vi "background2.vi"() -> ()   [LabVIEW 2014]
uses:
  <vilib>/Utility/inputDevices.llb/keyboardAcquire.vi
  <vilib>/Utility/inputDevices.llb/closeKeyboard.vi
panel:
  out "1jump":bool=TRUE
  out "black hole":T1
  out "火右飛 2":bool=TRUE
  out "火左飛 2":bool
  out "火左飛":bool
  out "1":T2
  out "火右飛":bool=TRUE
  out "2":T3
  out "2-1":T2
  out "2-2":T3
  in  "stop jump2":bool
  out "Position:Top 2":i32
  out "Position:Left 2":i32
  in  "stop jump1":bool
  out "人1":T4
  out "keys pressed":T5(array[ring])
  in  "right/left 2":bool
  in  "人2":bool
  in  "right/left":bool
  in  "人1":bool
  out "人2":T4
  out "Position:Top":i32
  out "Position:Left":i32
  in  "stop":bool
  # "W:17\nS:31\nA:30\nD:32"
  # "上:72\n下:80\n左:75\n右:77"
  # "17"
  # "48"
  # "587"
  # "168"
  # "523"
  # "623"
  # "678"
  # "334"
  # "288"
  # "408"
  # "1049"
  # "212"
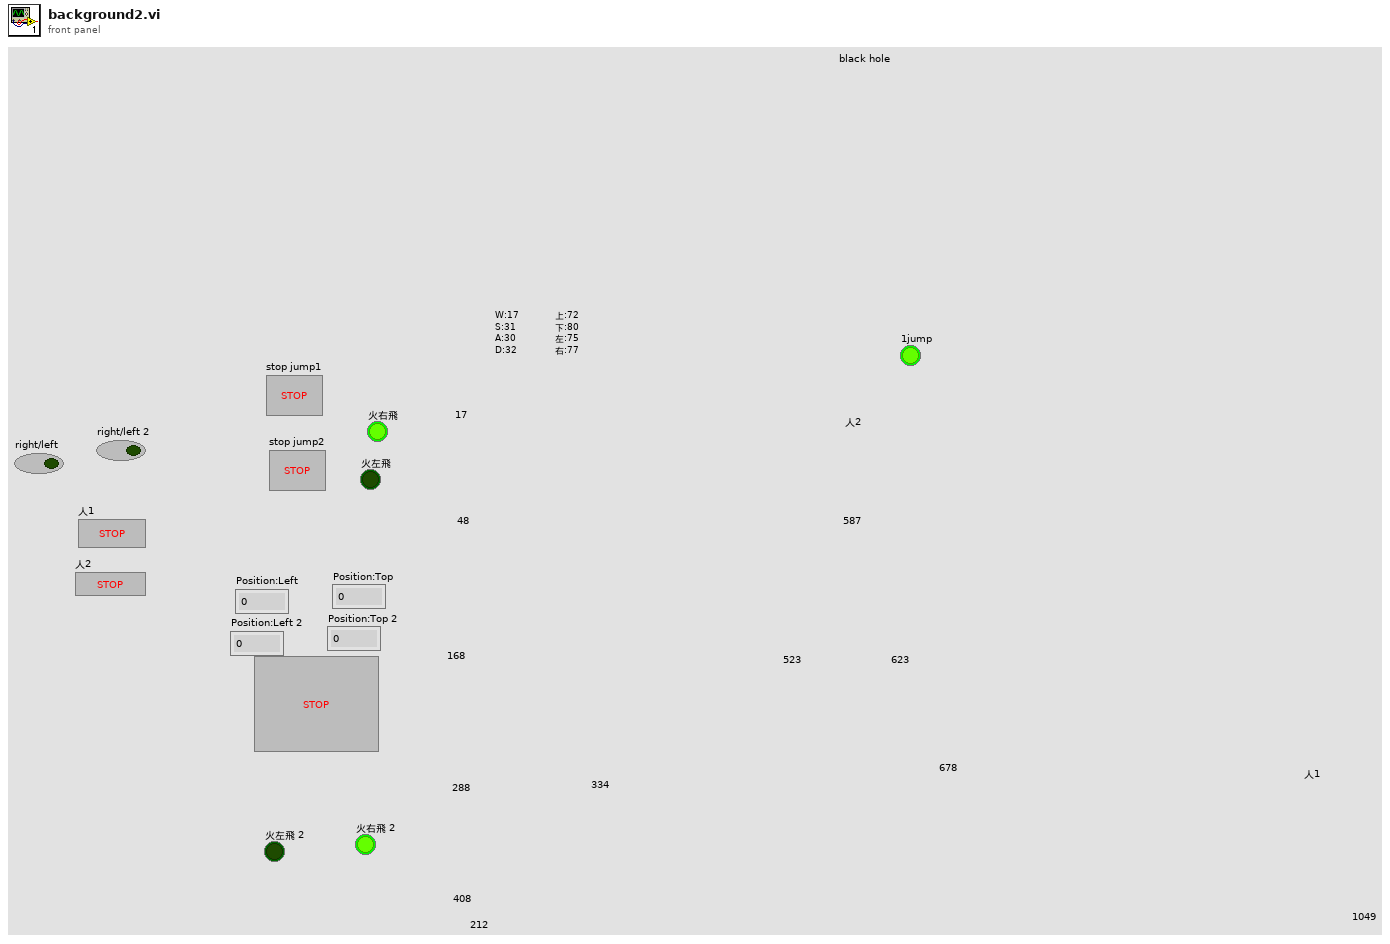
[diagram p1: front panel]
types:
  T1 = typedef "Control 4.ctl" = u16
  T2 = typedef "火焰.ctl" = u16
  T3 = typedef "火焰2.ctl" = u16
  T4 = typedef "Control 3.ctl" = u16
  T5 = enum16{"0", "1", "2", "3", "4", "5", "6", "7", "8", "9", "A", "B", "C", "D", "E", "F", "G", "H", "I", "J", "K", "L", "M", "N", "O", "P", "Q", "R", "S", "T", "U", "V", "W", "X", "Y", "Z", "F1", "F2", "F3", "F4", "F5", "F6", "F7", "F8", "F9", "F10", "F11", "F12", "F13", "F14", "F15", "ADD", "BACK", "BACKSLASH", "CAPITAL", "COMMA", "DECIMAL", "DELETE", "DIVIDE", "DOWN", "END", "EQUALS", "ESCAPE", "GRAVE (`)", "HOME", "INSERT", "LBRACKET", "LCONTROL", "LEFT", "L ALT", "LSHIFT", "LWIN", "MINUS", "MULTIPLY", "NEXT", "NUMLOCK", "NUMPAD_0", "NUMPAD_1", "NUMPAD_2", "NUMPAD_3", "NUMPAD_4", "NUMPAD_5", "NUMPAD_6", "NUMPAD_7", "NUMPAD_8", "NUMPAD_9", "PAUSE", "PERIOD", "PRIOR (PG UP)", "RBRACKET", "RCONTROL", "RETURN", "RIGHT", "R ALT", "RSHIFT", "RWIN", "SCROLL", "SEMICOLON", "SLASH", "SPACE", "SUBTRACT", "TAB", "UP", "ENTER (num pad)", "' (quote)"}[]
  T6 = enum16{"0", "1", "2", "3", "4", "5", "6", "7", "8", "9", "A", "B", "C", "D", "E", "F", "G", "H", "I", "J", "K", "L", "M", "N", "O", "P", "Q", "R", "S", "T", "U", "V", "W", "X", "Y", "Z", "F1", "F2", "F3", "F4", "F5", "F6", "F7", "F8", "F9", "F10", "F11", "F12", "F13", "F14", "F15", "ADD", "BACK", "BACKSLASH", "CAPITAL", "COMMA", "DECIMAL", "DELETE", "DIVIDE", "DOWN", "END", "EQUALS", "ESCAPE", "GRAVE (`)", "HOME", "INSERT", "LBRACKET", "LCONTROL", "LEFT", "L ALT", "LSHIFT", "LWIN", "MINUS", "MULTIPLY", "NEXT", "NUMLOCK", "NUMPAD_0", "NUMPAD_1", "NUMPAD_2", "NUMPAD_3", "NUMPAD_4", "NUMPAD_5", "NUMPAD_6", "NUMPAD_7", "NUMPAD_8", "NUMPAD_9", "PAUSE", "PERIOD", "PRIOR (PG UP)", "RBRACKET", "RCONTROL", "RETURN", "RIGHT", "R ALT", "RSHIFT", "RWIN", "SCROLL", "SEMICOLON", "SLASH", "SPACE", "SUBTRACT", "TAB", "UP", "ENTER (num pad)", "' (quote)"}
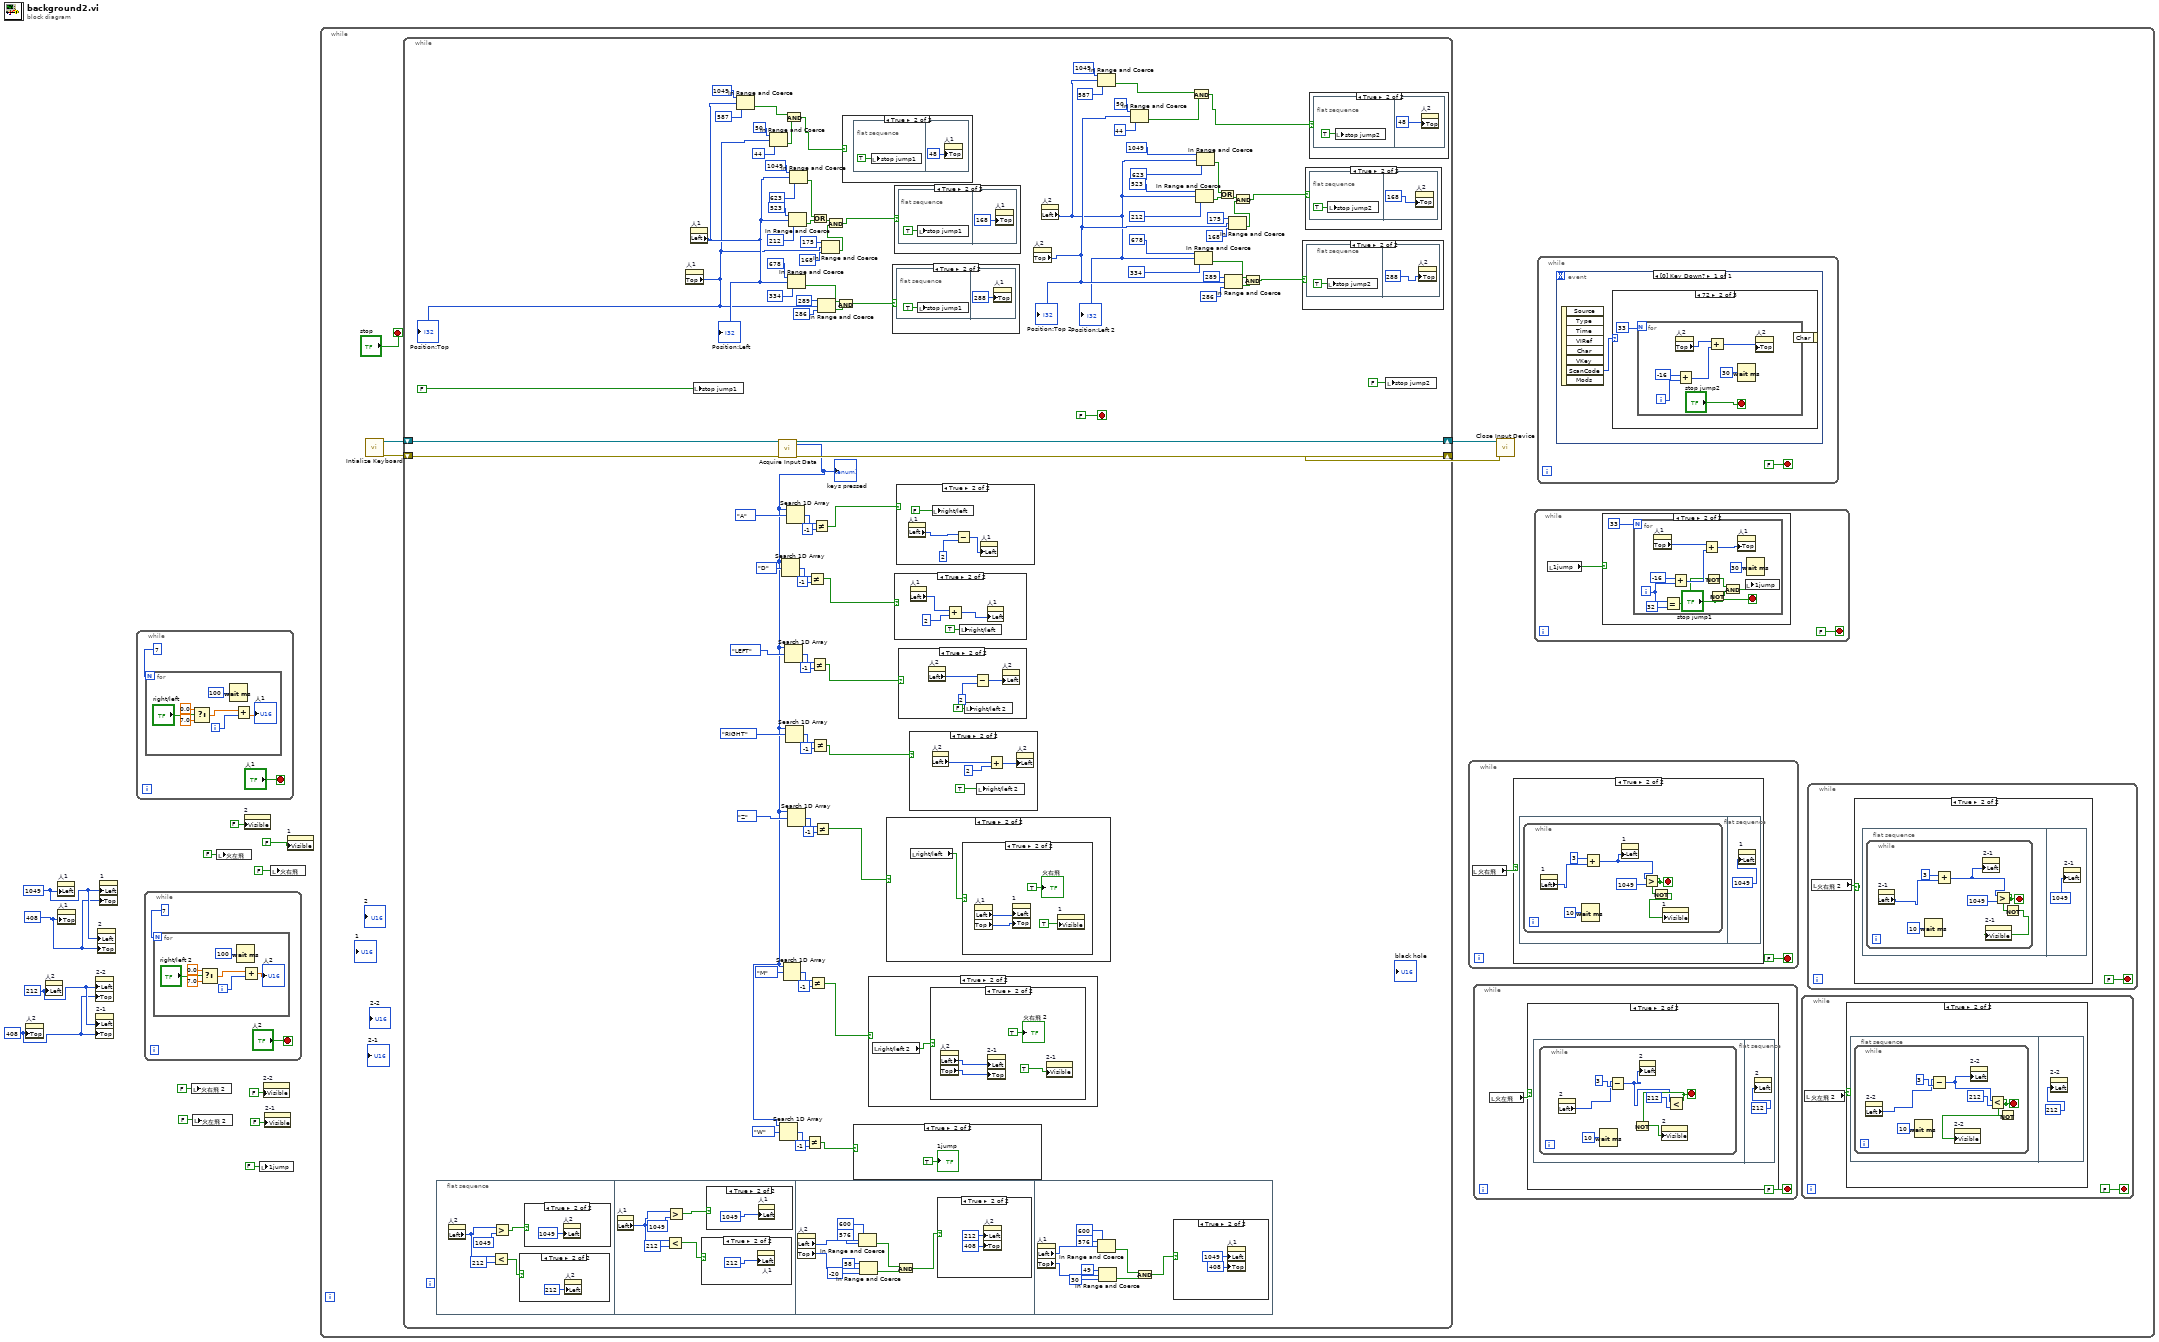
[diagram p0: block diagram]
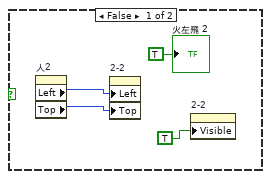
[diagram p17: hidden frame]
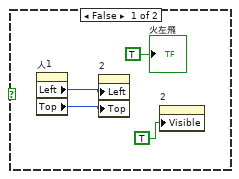
[diagram p19: hidden frame]
diagram:
  w2 = 408 ("Position:Top")
  w3 = 212 ("Position:Left")
  w4 = 408 ("Position:Top")
  w5 = 1049 ("Position:Left")
  n1 = property on="人2" class="Ring (strict)"("Top"=w2) -> ()  [unwired: 2 in, 2 out]
  n2 = property on="人2" class="Ring (strict)"("Left"=w3) -> ()  [unwired: 2 in, 2 out]
  n3 = property on="人1" class="Ring (strict)"("Left"=w5) -> ()  [unwired: 2 in, 2 out]
  n4 = property on="人1" class="Ring (strict)"("Top"=w4) -> ()  [unwired: 2 in, 2 out]
  n5 = property on="2-2" class="Ring (strict)"("Left"=w3, "Top"=w2) -> ()  [unwired: 2 in, 2 out]
  n6 = property on="2-1" class="Ring (strict)"("Left"=w3, "Top"=w2) -> ()  [unwired: 2 in, 2 out]
  n7 = property on="2" class="Ring (strict)"("Left"=w5, "Top"=w4) -> ()  [unwired: 2 in, 2 out]
  n8 = property on="1" class="Ring (strict)"("Left"=w5, "Top"=w4) -> ()  [unwired: 2 in, 2 out]
  n9 = while {
    stop <- "人1" stop-if-true
    n10 = for {
      N: 7 -> [_]
      i -> [w21]
      n11 = Select(t=0.0, s="right/left", f=7.0) -> (s? t:f=w18:dbl)
      n12 = Wait (ms)(milliseconds to wait=u32 100) -> ()  [unwired: 1 out]
      n13 = Add(x=w18, y=w21) -> (x+y=→"人1":dbl)
    }
  }
  n14 = while {
    stop <- "人2" stop-if-true
    n15 = for {
      N: 7 -> [_]
      i -> [w30]
      n16 = Select(t=0.0, s="right/left 2", f=7.0) -> (s? t:f=w28:dbl)
      n17 = Wait (ms)(milliseconds to wait=u32 100) -> ()  [unwired: 1 out]
      n18 = Add(x=w28, y=w30) -> (x+y=→"人2":dbl)
    }
  }
  n19 = local write "火右飛 2"(FALSE ("火右飛 2")) -> ()
  n20 = local write "火左飛 2"(FALSE ("火左飛 2")) -> ()
  n21 = local write "火左飛"(FALSE ("火左飛")) -> ()
  n22 = property on="2" class="Ring (strict)"("Visible"=FALSE) -> ()  [unwired: 2 in, 2 out]
  n23 = local write "1jump"(FALSE ("1jump")) -> ()
  n24 = property on="2-2" class="Ring (strict)"("Visible"=FALSE) -> ()  [unwired: 2 in, 2 out]
  n25 = property on="2-1" class="Ring (strict)"("Visible"=FALSE) -> ()  [unwired: 2 in, 2 out]
  n26 = local write "火右飛"(FALSE ("Boolean")) -> ()
  n27 = property on="1" class="Ring (strict)"("Visible"=FALSE) -> ()  [unwired: 2 in, 2 out]
  n28 = while {
    stop <- "stop" stop-if-true
    n29 = call <vilib>:"Intialize Keyboard.vi"() -> ("error out"=w34:errorcluster, "device ID"=w35:refnum<k1>)  [unwired: 10 in]
    n30 = while {
      shift-right: [w191] -> w32
      shift-left: w35 -> [w188]
      shift-right: [w190] -> w33
      shift-left: w34 -> [w189]
      stop <- FALSE stop-if-true
      n31 = flat-sequence {
        frame #0 {
          n32 = property on="人2" class="Ring (strict)"() -> ("Left"=w195:i32)  [unwired: 2 in, 2 out]
          n33 = Less?(x=w195, y=212) -> (x < y?=w192:bool)
          n34 = Greater?(x=w195, y=1049) -> (0:w193:bool)
          n35 = case shown="True" w192 {
            frame False {
            }
            frame True {
              n36 = property on="人2" class="Ring (strict)"("Left"=212 ("Position:Left")) -> ()  [unwired: 2 in, 2 out]
            }
          }
          n37 = case shown="True" w193 {
            frame False {
            }
            frame True {
              n38 = property on="人2" class="Ring (strict)"("Left"=1049 ("Position:Left")) -> ()  [unwired: 2 in, 2 out]
            }
          }
        }
        frame #1 {
          n39 = property on="人1" class="Ring (strict)"() -> ("Left"=w203:i32)  [unwired: 2 in, 2 out]
          n40 = Less?(x=w203, y=212) -> (x < y?=w202:bool)
          n41 = Greater?(x=w203, y=1049) -> (0:w201:bool)
          n42 = case shown="True" w202 {
            frame False {
            }
            frame True {
              n43 = property on="人1" class="Ring (strict)"("Left"=212 ("Position:Left")) -> ()  [unwired: 2 in, 2 out]
            }
          }
          n44 = case shown="True" w201 {
            frame False {
            }
            frame True {
              n45 = property on="人1" class="Ring (strict)"("Left"=1049 ("Position:Left")) -> ()  [unwired: 2 in, 2 out]
            }
          }
        }
        frame #2 {
          n46 = property on="人2" class="Ring (strict)"() -> ("Left"=w206:i32, "Top"=w209:i32)  [unwired: 2 in, 2 out]
          n47 = In Range and Coerce(upper limit=576, x=w206, lower limit=600) -> (In Range?=w213:bool)  [unwired: 1 out]
          n48 = In Range and Coerce(upper limit=58, x=w209, lower limit=-20) -> (In Range?=w212:bool)  [unwired: 1 out]
          n49 = And(x=w213, y=w212) -> (x .and. y?=w214:bool)
          n50 = case shown="True" w214 {
            frame False {
            }
            frame True {
              n51 = property on="人2" class="Ring (strict)"("Left"=212 ("Position:Left"), "Top"=408 ("Position:Top")) -> ()  [unwired: 2 in, 2 out]
            }
          }
        }
        frame #3 {
          n52 = property on="人1" class="Ring (strict)"() -> ("Left"=w223:i32, "Top"=w224:i32)  [unwired: 2 in, 2 out]
          n53 = In Range and Coerce(upper limit=576, x=w223, lower limit=600) -> (In Range?=w217:bool)  [unwired: 1 out]
          n54 = In Range and Coerce(upper limit=49, x=w224, lower limit=30) -> (In Range?=w218:bool)  [unwired: 1 out]
          n55 = And(x=w217, y=w218) -> (x .and. y?=w225:bool)
          n56 = case shown="True" w225 {
            frame False {
            }
            frame True {
              n57 = property on="人1" class="Ring (strict)"("Left"=1049 ("Position:Left"), "Top"=408 ("Position:Top")) -> ()  [unwired: 2 in, 2 out]
            }
          }
        }
      }
      n58 = property on="人1" class="Ring (strict)"() -> ("Top"=w150:i32)  [unwired: 2 in, 2 out]
      "Position:Top" <- w150
      n59 = property on="人1" class="Ring (strict)"() -> ("Left"=w153:i32)  [unwired: 2 in, 2 out]
      "Position:Left" <- w153
      n60 = local write "stop jump1"(FALSE ("stop jump1")) -> ()
      n61 = In Range and Coerce(upper limit=1049, x=w153, lower limit=587) -> (In Range?=w149:bool)  [unwired: 1 out]
      n62 = In Range and Coerce(upper limit=50, x=w150, lower limit=44) -> (In Range?=w154:bool)  [unwired: 1 out]
      n63 = call-poly <vilib>:"Acquire Input Data.vi"("device ID"=w188, "error in (no error)"=w189) -> ("device ID"=w191:refnum<k1>, "keys pressed"=w103:T5, "error out"=w190:errorcluster)  [unwired: 15 in]
      "keys pressed" <- w103
      n64 = Search 1D Array(1D array=w103, element=T6."W") -> (index of element=w105:i32)  [unwired: 1 in]
      n65 = Search 1D Array(1D array=w103, element=T6."D") -> (index of element=w182:i32)  [unwired: 1 in]
      n66 = Search 1D Array(1D array=w103, element=T6."M") -> (index of element=w112:i32)  [unwired: 1 in]
      n67 = Search 1D Array(1D array=w103, element=T6."LEFT") -> (index of element=w179:i32)  [unwired: 1 in]
      n68 = And(x=w149, y=w154) -> (x .and. y?=w145:bool)
      n69 = Search 1D Array(1D array=w103, element=T6."RIGHT") -> (index of element=w175:i32)  [unwired: 1 in]
      n70 = Search 1D Array(1D array=w103, element=T6."A") -> (index of element=w185:i32)  [unwired: 1 in]
      n71 = In Range and Coerce(upper limit=678, x=w153, lower limit=334) -> (In Range?=w151:bool)  [unwired: 1 out]
      n72 = Search 1D Array(1D array=w103, element=T6."Z") -> (index of element=w115:i32)  [unwired: 1 in]
      n73 = In Range and Coerce(upper limit=523, x=w153, lower limit=212) -> (In Range?=w148:bool)  [unwired: 1 out]
      n74 = In Range and Coerce(upper limit=1049, x=w153, lower limit=623) -> (In Range?=w152:bool)  [unwired: 1 out]
      n75 = Not Equal?(x=w105, y=-1) -> (x != y?=w102:bool)
      n76 = Not Equal?(x=w182, y=-1) -> (x != y?=w108:bool)
      n77 = Not Equal?(x=w112, y=-1) -> (x != y?=w110:bool)
      n78 = Not Equal?(x=w179, y=-1) -> (x != y?=w177:bool)
      n79 = Or(x=w152, y=w148) -> (x .or. y?=w159:bool)
      n80 = Not Equal?(x=w175, y=-1) -> (x != y?=w173:bool)
      n81 = Not Equal?(x=w185, y=-1) -> (x != y?=w109:bool)
      n82 = Not Equal?(x=w115, y=-1) -> (x != y?=w107:bool)
      n83 = In Range and Coerce(upper limit=289, x=w150, lower limit=286 ("y")) -> (In Range?=w171:bool)  [unwired: 1 out]
      n84 = In Range and Coerce(upper limit=175, x=w150, lower limit=168 ("y")) -> (In Range?=w163:bool)  [unwired: 1 out]
      n85 = And(x=w159, y=w163) -> (x .and. y?=w146:bool)
      n86 = And(x=w151, y=w171) -> (x .and. y?=w147:bool)
      n87 = case shown="True" w145 {
        frame False {
        }
        frame True {
          n88 = flat-sequence {
            frame #0 {
              n89 = local write "stop jump1"(TRUE ("stop jump1")) -> ()
            }
            frame #1 {
              n90 = property on="人1" class="Ring (strict)"("Top"=48 ("Position:Top")) -> ()  [unwired: 2 in, 2 out]
            }
          }
        }
      }
      n91 = case shown="True" w102 {
        frame False {
        }
        frame True {
          "1jump" <- TRUE
        }
      }
      n92 = case shown="True" w110 {
        frame False {
        }
        frame True {
          n93 = local read "right/left 2"() -> (w229:bool)
          n94 = case shown="True" w229 {
            frame False {
              n95 = property on="人2" class="Ring (strict)"() -> ("Left"=w232:i32, "Top"=w231:i32)  [unwired: 2 in, 2 out]
              n96 = property on="2-2" class="Ring (strict)"("Left"=w232, "Top"=w231) -> ()  [unwired: 2 in, 2 out]
              n97 = property on="2-2" class="Ring (strict)"("Visible"=TRUE) -> ()  [unwired: 2 in, 2 out]
              "火左飛 2" <- TRUE
            }
            frame True {
              n98 = property on="人2" class="Ring (strict)"() -> ("Left"=w236:i32, "Top"=w235:i32)  [unwired: 2 in, 2 out]
              n99 = property on="2-1" class="Ring (strict)"("Left"=w236, "Top"=w235) -> ()  [unwired: 2 in, 2 out]
              n100 = property on="2-1" class="Ring (strict)"("Visible"=TRUE) -> ()  [unwired: 2 in, 2 out]
              "火右飛 2" <- TRUE
            }
          }
        }
      }
      n101 = case shown="True" w107 {
        frame False {
        }
        frame True {
          n102 = local read "right/left"() -> (w238:bool)
          n103 = case shown="True" w238 {
            frame False {
              n104 = property on="人1" class="Ring (strict)"() -> ("Left"=w241:i32, "Top"=w240:i32)  [unwired: 2 in, 2 out]
              n105 = property on="2" class="Ring (strict)"("Left"=w241, "Top"=w240) -> ()  [unwired: 2 in, 2 out]
              n106 = property on="2" class="Ring (strict)"("Visible"=TRUE) -> ()  [unwired: 2 in, 2 out]
              "火左飛" <- TRUE
            }
            frame True {
              n107 = property on="人1" class="Ring (strict)"() -> ("Left"=w245:i32, "Top"=w244:i32)  [unwired: 2 in, 2 out]
              n108 = property on="1" class="Ring (strict)"("Left"=w245, "Top"=w244) -> ()  [unwired: 2 in, 2 out]
              n109 = property on="1" class="Ring (strict)"("Visible"=TRUE) -> ()  [unwired: 2 in, 2 out]
              "火右飛" <- TRUE
            }
          }
        }
      }
      n110 = case shown="True" w147 {
        frame False {
        }
        frame True {
          n111 = flat-sequence {
            frame #0 {
              n112 = local write "stop jump1"(TRUE ("stop jump1")) -> ()
            }
            frame #1 {
              n113 = property on="人1" class="Ring (strict)"("Top"=288 ("Position:Top")) -> ()  [unwired: 2 in, 2 out]
            }
          }
        }
      }
      n114 = case shown="True" w146 {
        frame False {
        }
        frame True {
          n115 = flat-sequence {
            frame #0 {
              n116 = local write "stop jump1"(TRUE ("stop jump1")) -> ()
            }
            frame #1 {
              n117 = property on="人1" class="Ring (strict)"("Top"=168 ("Position:Top")) -> ()  [unwired: 2 in, 2 out]
            }
          }
        }
      }
      n118 = case shown="True" w108 {
        frame False {
        }
        frame True {
          n119 = property on="人1" class="Ring (strict)"() -> ("Left"=w269:i32)  [unwired: 2 in, 2 out]
          n120 = Add(x=w269, y=2) -> (x+y=w268:i32)
          n121 = local write "right/left"(TRUE ("right/left")) -> ()
          n122 = property on="人1" class="Ring (strict)"("Left"=w268) -> ()  [unwired: 2 in, 2 out]
        }
      }
      n123 = case shown="True" w109 {
        frame False {
        }
        frame True {
          n124 = property on="人1" class="Ring (strict)"() -> ("Left"=w272:i32)  [unwired: 2 in, 2 out]
          n125 = local write "right/left"(FALSE ("人1 right 2")) -> ()
          n126 = Subtract(x=w272, y=2) -> (x-y=w271:i32)
          n127 = property on="人1" class="Ring (strict)"("Left"=w271) -> ()  [unwired: 2 in, 2 out]
        }
      }
      n128 = case shown="True" w177 {
        frame False {
        }
        frame True {
          n129 = property on="人2" class="Ring (strict)"() -> ("Left"=w265:i32)  [unwired: 2 in, 2 out]
          n130 = local write "right/left 2"(FALSE ("right/left")) -> ()
          n131 = Subtract(x=w265, y=2) -> (x-y=w264:i32)
          n132 = property on="人2" class="Ring (strict)"("Left"=w264) -> ()  [unwired: 2 in, 2 out]
        }
      }
      n133 = case shown="True" w173 {
        frame False {
        }
        frame True {
          n134 = property on="人2" class="Ring (strict)"() -> ("Left"=w261:i32)  [unwired: 2 in, 2 out]
          n135 = local write "right/left 2"(TRUE ("人1 right 2")) -> ()
          n136 = Add(x=w261, y=2) -> (x+y=w260:i32)
          n137 = property on="人2" class="Ring (strict)"("Left"=w260) -> ()  [unwired: 2 in, 2 out]
        }
      }
      n138 = property on="人2" class="Ring (strict)"() -> ("Top"=w119:i32)  [unwired: 2 in, 2 out]
      "Position:Top 2" <- w119
      n139 = property on="人2" class="Ring (strict)"() -> ("Left"=w118:i32)  [unwired: 2 in, 2 out]
      "Position:Left 2" <- w118
      n140 = In Range and Coerce(upper limit=1049, x=w118, lower limit=587) -> (In Range?=w124:bool)  [unwired: 1 out]
      n141 = In Range and Coerce(upper limit=50, x=w119, lower limit=44) -> (In Range?=w127:bool)  [unwired: 1 out]
      n142 = And(x=w124, y=w127) -> (x .and. y?=w120:bool)
      n143 = In Range and Coerce(upper limit=678, x=w118, lower limit=334) -> (In Range?=w125:bool)  [unwired: 1 out]
      n144 = In Range and Coerce(upper limit=523, x=w118, lower limit=212) -> (In Range?=w123:bool)  [unwired: 1 out]
      n145 = In Range and Coerce(upper limit=1049, x=w118, lower limit=623) -> (In Range?=w126:bool)  [unwired: 1 out]
      n146 = Or(x=w126, y=w123) -> (x .or. y?=w132:bool)
      n147 = In Range and Coerce(upper limit=289, x=w119, lower limit=286 ("y")) -> (In Range?=w143:bool)  [unwired: 1 out]
      n148 = In Range and Coerce(upper limit=175, x=w119, lower limit=168 ("y")) -> (In Range?=w135:bool)  [unwired: 1 out]
      n149 = And(x=w132, y=w135) -> (x .and. y?=w121:bool)
      n150 = And(x=w125, y=w143) -> (x .and. y?=w122:bool)
      n151 = case shown="True" w122 {
        frame False {
        }
        frame True {
          n152 = flat-sequence {
            frame #0 {
              n153 = local write "stop jump2"(TRUE ("stop jump1")) -> ()
            }
            frame #1 {
              n154 = property on="人2" class="Ring (strict)"("Top"=288 ("Position:Top")) -> ()  [unwired: 2 in, 2 out]
            }
          }
        }
      }
      n155 = case shown="True" w121 {
        frame False {
        }
        frame True {
          n156 = flat-sequence {
            frame #0 {
              n157 = local write "stop jump2"(TRUE ("stop jump1")) -> ()
            }
            frame #1 {
              n158 = property on="人2" class="Ring (strict)"("Top"=168 ("Position:Top")) -> ()  [unwired: 2 in, 2 out]
            }
          }
        }
      }
      n159 = case shown="True" w120 {
        frame False {
        }
        frame True {
          n160 = flat-sequence {
            frame #0 {
              n161 = local write "stop jump2"(TRUE ("stop jump1")) -> ()
            }
            frame #1 {
              n162 = property on="人2" class="Ring (strict)"("Top"=48 ("Position:Top")) -> ()  [unwired: 2 in, 2 out]
            }
          }
        }
      }
      n163 = local write "stop jump2"(FALSE ("stop jump1 2")) -> ()
    }
    n164 = while {
      stop <- FALSE stop-if-true
      n165 = local read "火右飛"() -> (w73:bool)
      n166 = case shown="True" w73 {
        frame False {
        }
        frame True {
          n167 = flat-sequence {
            frame #0 {
              n168 = while {
                stop <- w78 stop-if-true
                n169 = property on="1" class="Ring (strict)"() -> ("Left"=w77:i32)  [unwired: 2 in, 2 out]
                n170 = Wait (ms)(milliseconds to wait=u32 10) -> ()  [unwired: 1 out]
                n171 = Add(x=3, y=w77) -> (x+y=w76:i32)
                n172 = property on="1" class="Ring (strict)"("Left"=w76) -> ()  [unwired: 2 in, 2 out]
                n173 = Greater?(x=w76, y=1049) -> (0:w78:bool)
                n174 = Not(x=w78) -> (.not. x?=w75:bool)
                n175 = property on="1" class="Ring (strict)"("Visible"=w75) -> ()  [unwired: 2 in, 2 out]
              }
            }
            frame #1 {
              n176 = property on="1" class="Ring (strict)"("Left"=1049 ("y")) -> ()  [unwired: 2 in, 2 out]
            }
          }
        }
      }
    }
    n177 = while {
      stop <- FALSE stop-if-true
      n178 = local read "火左飛"() -> (w83:bool)
      n179 = case shown="True" w83 {
        frame False {
        }
        frame True {
          n180 = flat-sequence {
            frame #0 {
              n181 = while {
                stop <- w90 stop-if-true
                n182 = property on="2" class="Ring (strict)"() -> ("Left"=w87:i32)  [unwired: 2 in, 2 out]
                n183 = Wait (ms)(milliseconds to wait=u32 10) -> ()  [unwired: 1 out]
                n184 = Subtract(x=w87, y=3 ("x")) -> (x-y=w84:i32)
                n185 = property on="2" class="Ring (strict)"("Left"=w84) -> ()  [unwired: 2 in, 2 out]
                n186 = Less?(x=w84, y=212) -> (x < y?=w90:bool)
                n187 = Not(x=w90) -> (.not. x?=w89:bool)
                n188 = property on="2" class="Ring (strict)"("Visible"=w89) -> ()  [unwired: 2 in, 2 out]
              }
            }
            frame #1 {
              n189 = property on="2" class="Ring (strict)"("Left"=212 ("y")) -> ()  [unwired: 2 in, 2 out]
            }
          }
        }
      }
    }
    n190 = call-poly <vilib>:"Close Input Device.vi"("error in (no error)"=w33, "device ID"=w32) -> ()  [unwired: 8 in, 1 out]
    n191 = while {
      stop <- FALSE stop-if-true
      n192 = local read "1jump"() -> (w37:bool)
      n193 = case shown="True" w37 {
        frame False {
        }
        frame True {
          n194 = for {
            N: 33 -> [_]
            i -> [w45]
            stop <- "stop jump1" stop-if-true
            n195 = property on="人1" class="Ring (strict)"() -> ("Top"=w48:i32)  [unwired: 2 in, 2 out]
            n196 = Equal?(x=w45, y=32) -> (x = y?=w43:bool)
            n197 = Add(x=-16, y=w45) -> (x+y=w50:i32)
            n198 = Add(x=w48, y=w50) -> (x+y=w47:i32)
            n199 = Not(x=w43) -> (.not. x?=w42:bool)
            n200 = Not(x="stop jump1") -> (.not. x?=w41:bool)
            n201 = And(x=w42, y=w41) -> (x .and. y?=w40:bool)
            n202 = property on="人1" class="Ring (strict)"("Top"=w47) -> ()  [unwired: 2 in, 2 out]
            n203 = local write "1jump"(w40) -> ()
            n204 = Wait (ms)(milliseconds to wait=u32 30) -> ()  [unwired: 1 out]
          }
        }
      }
    }
    n205 = while {
      stop <- FALSE stop-if-true
      n206 = event shown="[0] Key Down?" {
        selector: _ -> [_]
        dyn-events: _ -> [_]
        timeout: _ -> [_]
        event Key Down? {
          n207 = event-data() -> ("ScanCode"=w93:i16)  [unwired: 1 in, 7 out]
          n208 = case shown="72" w93 {
            frame Default {
            }
            frame 72 {
              n209 = for {
                N: 33 -> [_]
                i -> [w101]
                stop <- "stop jump2" stop-if-true
                n210 = property on="人2" class="Ring (strict)"() -> ("Top"=w97:i32)  [unwired: 2 in, 2 out]
                n211 = Add(x=-16, y=w101) -> (x+y=w99:i32)
                n212 = Add(x=w97, y=w99) -> (x+y=w96:i32)
                n213 = Wait (ms)(milliseconds to wait=u32 30) -> ()  [unwired: 1 out]
                n214 = property on="人2" class="Ring (strict)"("Top"=w96) -> ()  [unwired: 2 in, 2 out]
              }
            }
            frame 17 {
            }
          }
          n215 = event-data() -> ()  [unwired: 2 in, 1 out]
        }
      }
    }
    n216 = while {
      stop <- FALSE stop-if-true
      n217 = local read "火左飛 2"() -> (w53:bool)
      n218 = case shown="True" w53 {
        frame False {
        }
        frame True {
          n219 = flat-sequence {
            frame #0 {
              n220 = while {
                stop <- w60 stop-if-true
                n221 = property on="2-2" class="Ring (strict)"() -> ("Left"=w57:i32)  [unwired: 2 in, 2 out]
                n222 = Wait (ms)(milliseconds to wait=u32 10) -> ()  [unwired: 1 out]
                n223 = Subtract(x=w57, y=3 ("x")) -> (x-y=w54:i32)
                n224 = property on="2-2" class="Ring (strict)"("Left"=w54) -> ()  [unwired: 2 in, 2 out]
                n225 = Less?(x=w54, y=212) -> (x < y?=w60:bool)
                n226 = Not(x=w60) -> (.not. x?=w59:bool)
                n227 = property on="2-2" class="Ring (strict)"("Visible"=w59) -> ()  [unwired: 2 in, 2 out]
              }
            }
            frame #1 {
              n228 = property on="2-2" class="Ring (strict)"("Left"=212 ("y")) -> ()  [unwired: 2 in, 2 out]
            }
          }
        }
      }
    }
    n229 = while {
      stop <- FALSE stop-if-true
      n230 = local read "火右飛 2"() -> (w63:bool)
      n231 = case shown="True" w63 {
        frame False {
        }
        frame True {
          n232 = flat-sequence {
            frame #0 {
              n233 = while {
                stop <- w68 stop-if-true
                n234 = property on="2-1" class="Ring (strict)"() -> ("Left"=w67:i32)  [unwired: 2 in, 2 out]
                n235 = Wait (ms)(milliseconds to wait=u32 10) -> ()  [unwired: 1 out]
                n236 = Add(x=3, y=w67) -> (x+y=w66:i32)
                n237 = property on="2-1" class="Ring (strict)"("Left"=w66) -> ()  [unwired: 2 in, 2 out]
                n238 = Greater?(x=w66, y=1049) -> (0:w68:bool)
                n239 = Not(x=w68) -> (.not. x?=w65:bool)
                n240 = property on="2-1" class="Ring (strict)"("Visible"=w65) -> ()  [unwired: 2 in, 2 out]
              }
            }
            frame #1 {
              n241 = property on="2-1" class="Ring (strict)"("Left"=1049 ("y")) -> ()  [unwired: 2 in, 2 out]
            }
          }
        }
      }
    }
  }
